vi "Database Test Null.vi"() -> ()   [LabVIEW 2018]
doc: "This example demonstrates how to verify whether a variant in the database is Null or not. This example first inserts two Null values and some numeric and string values to the database. This example then uses the Database Variant To Data function to display these values and uses the DB Tools Null VI to verify whether the value is Null or not."
uses:
  <vilib>/addons/database/Auxilliary.llb/DB Tools Column Info.ctl
  <vilib>/addons/database/Auxilliary.llb/DB Tools DataTypes.ctl
  <vilib>/addons/database/Auxilliary.llb/DB Tools Parameter Info.ctl
  <vilib>/addons/database/Auxilliary.llb/DB Tools Parameter Dir.ctl
  <vilib>/addons/database/Connection.llb/DB Tools Open Connec (Path).vi
  <vilib>/addons/database/Command.llb/Cmd Set Parameter Value (C).vi
  <vilib>/addons/database/Command.llb/Cmd Execute.vi
  <vilib>/addons/database/Recordset.llb/Rec Destroy - Command.vi
  <vilib>/addons/database/Command.llb/Cmd Delete.vi
  <vilib>/addons/database/Connection.llb/Conn Execute.vi
  <vilib>/addons/database/Recordset.llb/Rec Destroy - Connection.vi
  <vilib>/addons/database/_DB Variant To Data/Database Variant To Data.xnode
  <vilib>/addons/database/NI_Database_API.lvlib
panel:
  out "Value":string[][](array[string])
  out "Value is NULL?":bool[][](array[boolean])
  # "Overview: Demonstrates how to verify whether or not a database table value is NULL.\nRequirements: Database Connectivity Toolkit\nInstructions:\nRun the VI. The Value is NULL? array will indicate which items in the Value table are NULL values."
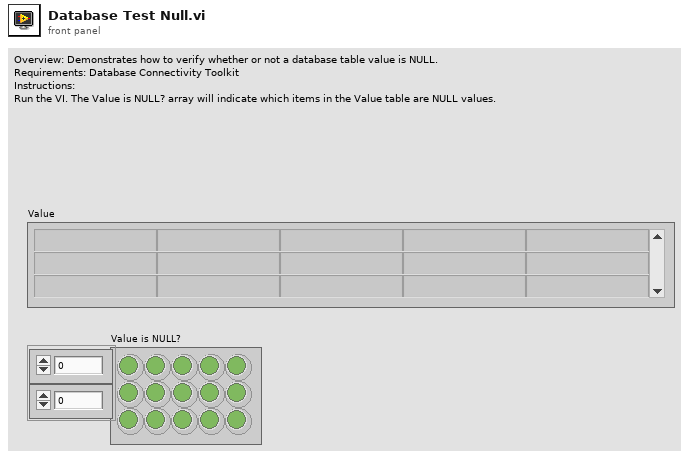
[diagram p1: front panel]
types:
  T1 = typedef "NI_Database_API.lvlib/DB Tools Parameter Info.ctl" = cluster{"parameter name":string, "type":T2, "direction":T3, "value":variant}
  T2 = typedef "NI_Database_API.lvlib/DB Tools DataTypes.ctl" = enum16{"String", "Long (I32)", "Single (SGL)", "Double (DBL)", "Date/Time", "Binary"}
  T3 = typedef "NI_Database_API.lvlib/DB Tools Parameter Dir.ctl" = enum32{"Input", "Output", "Input/Output", "Return Value"}
  T4 = typedef "NI_Database_API.lvlib/DB Tools Column Info.ctl" = cluster{"column name":string, "data type":T2, "size":i32, "allow null?":bool}
  T5 = typedef "NI_Database_API.lvlib/Conn ObjectReference.ctl" = refnum<k1>
  T6 = typedef "NI_Database_API.lvlib/Cmd ObjectReference.ctl" = refnum<k1>
  T7 = typedef "NI_Database_API.lvlib/Cmd-Rec Object Reference.ctl" = refnum<k1>
  T8 = typedef "NI_Database_API.lvlib/Rec ObjectReference.ctl" = refnum<k1>
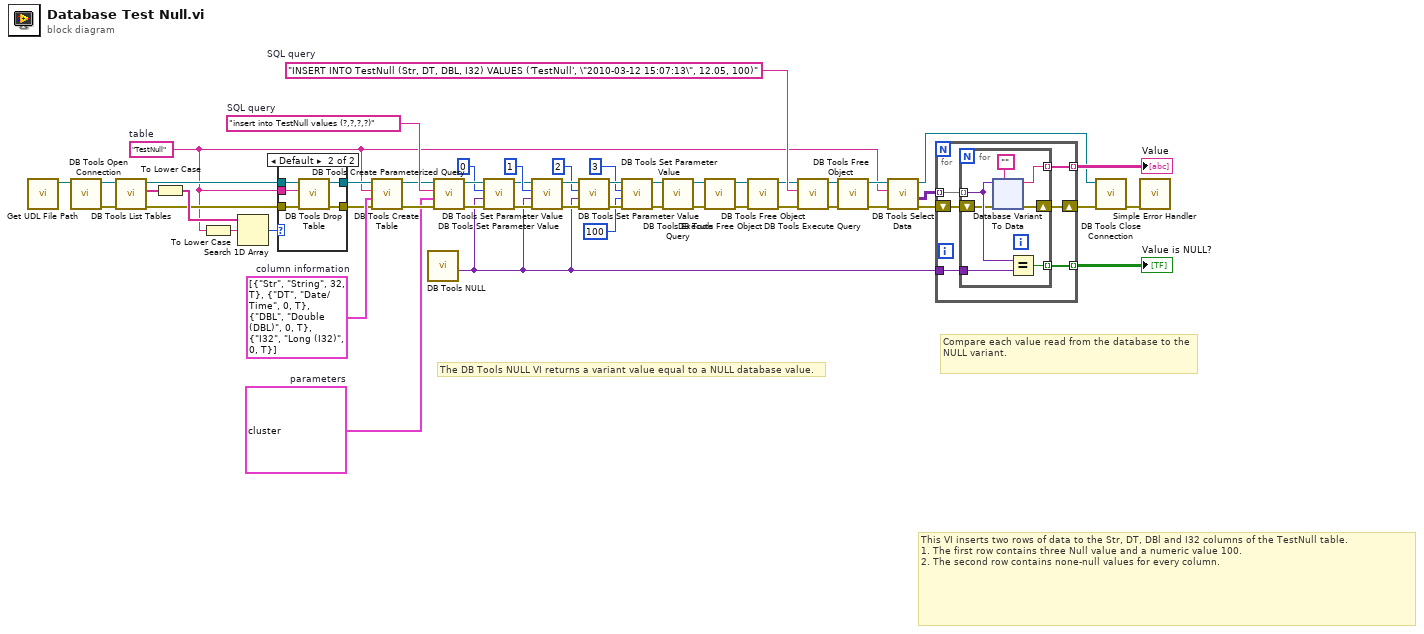
[diagram p0: block diagram]
diagram:
  w12 = T1[] [{"parameter name"="Str", "type"=enum."String", "direction"=enum."Input", "value"=variant}, {"parameter name"="DT", "type"=enum."Date/Time", "direction"=enum."Input", "value"=variant}, {"parameter name"="DBL", "type"=enum."Double (DBL)", "direction"=enum."Input", "value"=variant}, {"parameter name"="I32", "type"=enum."Long (I32)", "direction"=enum."Input", "value"=variant}]  # parameters
  w43 = T4[] [{"column name"="Str", "data type"=enum."String", "size"=32, "allow null?"=TRUE}, {"column name"="DT", "data type"=enum."Date/Time", "size"=0, "allow null?"=TRUE}, {"column name"="DBL", "data type"=enum."Double (DBL)", "size"=0, "allow null?"=TRUE}, {"column name"="I32", "data type"=enum."Long (I32)", "size"=0, "allow null?"=TRUE}]  # column information
  w32 = "insert into TestNull values (?,?,?,?)"  # SQL query
  w2 = "TestNull"  # table
  w47 = "INSERT INTO TestNull (Str, DT, DBL, I32) VALUES ('TestNull', \"2010-03-12 15:07:13\", 12.05, 100)"  # SQL query
  # "Compare each value read from the database to the NULL variant."
  # "The DB Tools NULL VI returns a variant value equal to a NULL database value."
  # "This VI inserts two rows of data to the Str, DT, DBl and I32 columns of the TestNull table. \n1. The first row contains three Null value and a numeric value 100. \n2. The second row contains none-null values for every column."
  n1 = call "Get UDL File Path.vi"() -> ("UDL file path"=w49:path)  [unwired: 11 in]
  n2 = call-poly <vilib>:"DB Tools Open Connection.vi"("connection information"=w49) -> ("error out"=w50:errorcluster, "connection reference"=w51:T5)  [unwired: 7 in]
  n3 = call <vilib>:"DB Tools List Tables.vi"("error in (no error)"=w50, "connection reference"=w51) -> ("error out"=w24:errorcluster, "tables"=w23:string[], "connection reference out"=w25:T5)  [unwired: 3 in]
  n4 = To Lower Case(string=w23) -> (all lower case string=w26:string[])
  n5 = To Lower Case(string=w2) -> (all lower case string=w27:string)
  n6 = Search 1D Array(1D array=w26, element=w27) -> (index of element=w28:i32)  [unwired: 1 in]
  n7 = case shown="Default" w28 {
    tunnel: w24 -> [w52 w58]
    tunnel: w25 -> [w53 w57]
    tunnel: [w53 w56] -> w30
    tunnel: [w52 w55] -> w29
    tunnel: w2 -> [_ w54]
    frame -1 {
    }
    frame Default {
      n8 = call <vilib>:"DB Tools Drop Table.vi"("error in (no error)"=w58, "table"=w54, "connection reference"=w57) -> ("error out"=w55:errorcluster, "connection reference out"=w56:T5)  [unwired: 5 in]
    }
  }
  n9 = call <vilib>:"DB Tools Create Table.vi"("error in (no error)"=w29, "column information"=w43, "table"=w2, "connection reference"=w30) -> ("error out"=w38:errorcluster, "connection reference out"=w31:T5)  [unwired: 4 in]
  n10 = call <vilib>:"DB Tools NULL.vi"() -> ("NULL"=w1:variant)  [unwired: 10 in, 1 out]
  n11 = call <vilib>:"DB Tools Create Parameterized Query.vi"("error in (no error)"=w38, "parameters"=w12, "SQL query"=w32, "connection reference"=w31) -> ("error out"=w41:errorcluster, "command reference"=w42:T6)  [unwired: 2 in, 2 out]
  n12 = call-poly <vilib>:"DB Tools Set Parameter Value.vi"("error in (no error)"=w41, "value"=w1, "parameter index"=0, "command reference"=w42) -> ("error out"=w33:errorcluster, "command reference out"=w34:T6)  [unwired: 4 out]
  n13 = call-poly <vilib>:"DB Tools Set Parameter Value.vi"("error in (no error)"=w33, "value"=w1, "parameter index"=1, "command reference"=w34) -> ("error out"=w16:errorcluster, "command reference out"=w15:T6)  [unwired: 4 out]
  n14 = call-poly <vilib>:"DB Tools Set Parameter Value.vi"("error in (no error)"=w16, "value"=w1, "parameter index"=2, "command reference"=w15) -> ("error out"=w17:errorcluster, "command reference out"=w18:T6)  [unwired: 4 out]
  n15 = call-poly <vilib>:"DB Tools Set Parameter Value.vi"("error in (no error)"=w17, "value"=100, "parameter index"=3, "command reference"=w18) -> ("error out"=w20:errorcluster, "command reference out"=w19:T6)  [unwired: 4 out]
  n16 = call-poly <vilib>:"DB Tools Execute Query.vi"("error in (no error)"=w20, "command reference"=w19) -> ("error out"=w35:errorcluster, "command-recordset reference"=w36:T7)  [unwired: 2 in, 4 out]
  n17 = call-poly <vilib>:"DB Tools Free Object.vi"("error in (no error)"=w35, "command-recordset reference"=w36) -> ("error out"=w37:errorcluster, "command reference"=w44:T6)  [unwired: 8 out]
  n18 = call-poly <vilib>:"DB Tools Free Object.vi"("error in (no error)"=w37, "command reference"=w44) -> ("error out"=w21:errorcluster, "connection reference"=w22:T5)  [unwired: 8 out]
  n19 = call-poly <vilib>:"DB Tools Execute Query.vi"("error in (no error)"=w21, "SQL query"=w47, "connection reference"=w22) -> ("error out"=w46:errorcluster, "recordset reference"=w45:T8)  [unwired: 1 in, 4 out]
  n20 = call-poly <vilib>:"DB Tools Free Object.vi"("error in (no error)"=w46, "recordset reference"=w45) -> ("error out"=w5:errorcluster, "connection reference"=w6:T5)  [unwired: 8 out]
  n21 = call <vilib>:"DB Tools Select Data.vi"("error in (no error)"=w5, "table"=w2, "connection reference"=w6) -> ("error out"=w7:errorcluster, "data"=w10:variant[][], "connection reference out"=w4:T5)  [unwired: 1 in, 2 out]
  n22 = for {
    tunnel: w10 -> [w64] mode=indexing
    tunnel: [w63] -> w9 mode=indexing
    tunnel: [w62] -> w8 mode=indexing
    shift-right: [w60] -> w3
    shift-left: w7 -> [w61]
    tunnel: w1 -> [w59]
    n23 = for {
      tunnel: w64 -> [w67] mode=indexing
      tunnel: [w70] -> w63 mode=indexing
      tunnel: [w69] -> w62 mode=indexing
      shift-right: [w65] -> w60
      shift-left: w61 -> [w66]
      tunnel: w59 -> [w68]
      n24 = xnode "Database Variant To Data"("database variant"=w67, "error in"=w66, "type"="") -> ("data"=w70:string, "error out"=w65:errorcluster)
      n25 = Equal?(x=w67, y=w68) -> (x = y?=w69:bool)
    }
  }
  "Value" <- w9
  "Value is NULL?" <- w8
  n26 = call <vilib>:"DB Tools Close Connection.vi"("error in (no error)"=w3, "connection reference"=w4) -> ("error out"=w48:errorcluster)  [unwired: 5 out]
  n27 = call <vilib>:"Simple Error Handler.vi"("error in (no error)"=w48) -> ()  [unwired: 4 in, 5 out]
